vi "Positions2.0.vi"() -> ()   [LabVIEW 2014]
panel:
  in  "Position":enum16{"0", "1", "2", "3", "4"}(ring)
  out "Direction":enum16{"stop", "up", "down"}(ring)=enum."up"
  out "Current Position":i32
  in  "distance traveled":i32
  in  "Distance 5":dbl
  in  "Distance 4":dbl
  in  "Distance 3":dbl
  in  "Distance 2":dbl
  in  "Distance 1":dbl
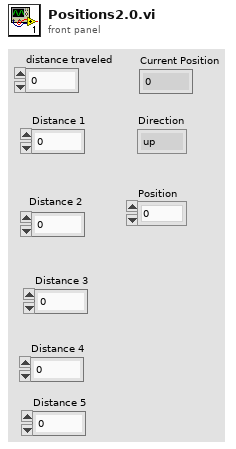
[diagram p1: front panel]
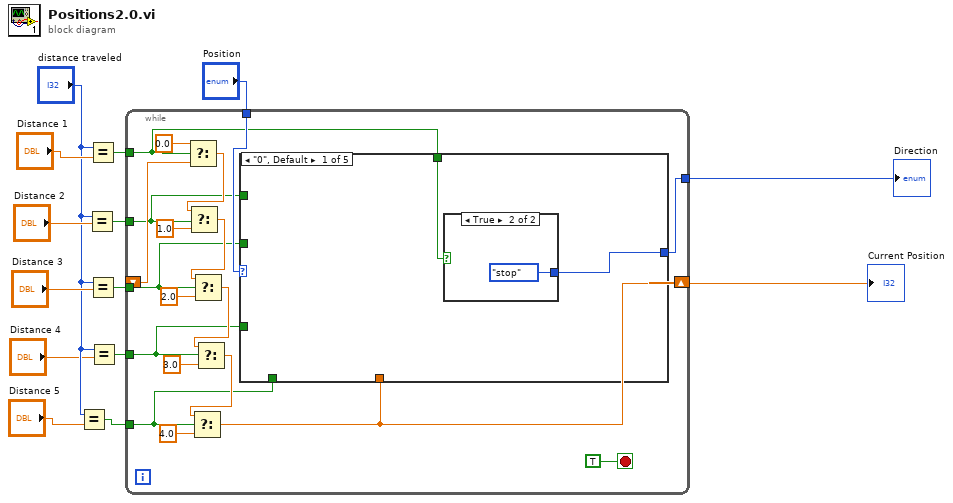
[diagram p0: block diagram]
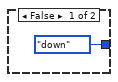
[diagram p2: hidden frame]
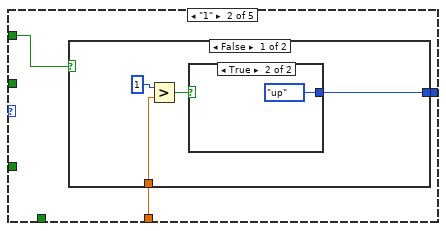
[diagram p3: hidden frame]
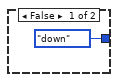
[diagram p4: hidden frame]
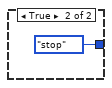
[diagram p5: hidden frame]
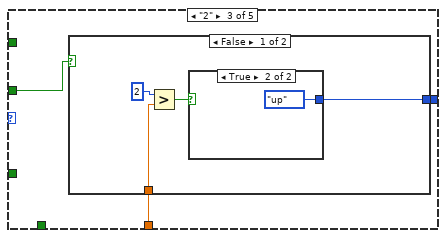
[diagram p6: hidden frame]
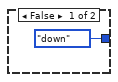
[diagram p7: hidden frame]
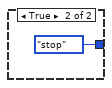
[diagram p8: hidden frame]
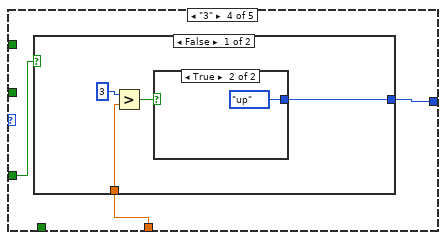
[diagram p9: hidden frame]
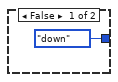
[diagram p10: hidden frame]
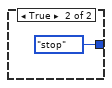
[diagram p11: hidden frame]
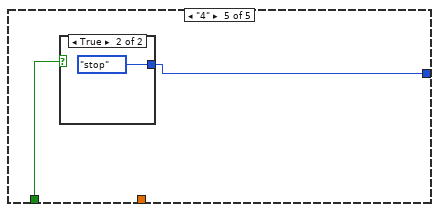
[diagram p12: hidden frame]
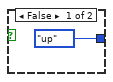
[diagram p13: hidden frame]
diagram:
  n1 = Equal?(x="distance traveled", y="Distance 5") -> (x = y?=w4:bool)
  n2 = Equal?(x="distance traveled", y="Distance 2") -> (x = y?=w7:bool)
  n3 = Equal?(x="distance traveled", y="Distance 1") -> (x = y?=w13:bool)
  n4 = Equal?(x="distance traveled", y="Distance 3") -> (x = y?=w6:bool)
  n5 = Equal?(x="distance traveled", y="Distance 4") -> (x = y?=w5:bool)
  n6 = while {
    tunnel: w13 -> [w19]
    tunnel: w7 -> [w18]
    tunnel: w6 -> [w17]
    tunnel: w5 -> [w16]
    tunnel: w4 -> [w15]
    shift-right: [w20] -> w3
    shift-left: _ -> [w27]
    tunnel: [w22] -> w2
    tunnel: "Position" -> [w21]
    stop <- TRUE stop-if-true
    n7 = Select(t=0.0, s=w19, f=w27) -> (s? t:f=w32:dbl)
    n8 = Select(t=w32, s=w18, f=1.0) -> (s? t:f=w31:dbl)
    n9 = Select(t=w31, s=w17, f=2.0) -> (s? t:f=w30:dbl)
    n10 = Select(t=w30, s=w16, f=3.0) -> (s? t:f=w29:dbl)
    n11 = Select(t=w29, s=w15, f=4.0) -> (s? t:f=w20:dbl)
    n12 = case shown="\"0\", Default" w21 {
      tunnel: [w35 w40 w50 w60 w69] -> w22
      tunnel: w20 -> [_ w39 w49 w59 _]
      tunnel: w19 -> [w34 _ _ _ _]
      tunnel: w18 -> [_ w38 _ _ _]
      tunnel: w17 -> [_ _ w48 _ _]
      tunnel: w16 -> [_ _ _ w58 _]
      tunnel: w15 -> [_ _ _ _ w68]
      frame "0", Default {
        n13 = case shown="True" w34 {
          tunnel: [enum16{"stop", "up", "down"}."down" ("Direction") enum16{"stop", "up", "down"}."stop" ("Direction")] -> w35
          frame False {
          }
          frame True {
          }
        }
      }
      frame "1" {
        n14 = case shown="False" w38 {
          tunnel: [w44 enum16{"stop", "up", "down"}."stop" ("Direction")] -> w40
          tunnel: w39 -> [w41 _]
          frame False {
            n15 = Greater?(x=1, y=w41) -> (0:w42:bool)
            n16 = case shown="True" w42 {
              tunnel: [enum16{"stop", "up", "down"}."down" ("Direction") enum16{"stop", "up", "down"}."up" ("Direction")] -> w44
              frame False {
              }
              frame True {
              }
            }
          }
          frame True {
          }
        }
      }
      frame "2" {
        n17 = case shown="False" w48 {
          tunnel: [w54 enum16{"stop", "up", "down"}."stop" ("Direction")] -> w50
          tunnel: w49 -> [w51 _]
          frame False {
            n18 = Greater?(x=2, y=w51) -> (0:w53:bool)
            n19 = case shown="True" w53 {
              tunnel: [enum16{"stop", "up", "down"}."down" ("Direction") enum16{"stop", "up", "down"}."up" ("Direction")] -> w54
              frame False {
              }
              frame True {
              }
            }
          }
          frame True {
          }
        }
      }
      frame "3" {
        n20 = case shown="False" w58 {
          tunnel: [w64 enum16{"stop", "up", "down"}."stop" ("Direction")] -> w60
          tunnel: w59 -> [w61 _]
          frame False {
            n21 = Greater?(x=3, y=w61) -> (0:w63:bool)
            n22 = case shown="True" w63 {
              tunnel: [enum16{"stop", "up", "down"}."down" ("Direction") enum16{"stop", "up", "down"}."up" ("Direction")] -> w64
              frame False {
              }
              frame True {
              }
            }
          }
          frame True {
          }
        }
      }
      frame "4" {
        n23 = case shown="True" w68 {
          tunnel: [enum16{"stop", "up", "down"}."up" ("Direction") enum16{"stop", "up", "down"}."stop" ("Direction")] -> w69
          frame False {
          }
          frame True {
          }
        }
      }
    }
  }
  "Current Position" <- w3
  "Direction" <- w2
